vi "VNA Calibration - SParam.vi"(8 "error in":errorcluster, 10 "RFmxVNA Settings":T1={"Resource Name"="", "vCal Name"="", "RFmxVNA Calset Enable"=FALSE, "RFmxVNA Calset Interpolation"=FALSE, "Calset File Path"="", "RFmxVNA attenuation mode"=enum."s2p File", "RFmxVNA Port1 s2p file path"="", "RFmxVNA Port1 s-parameters orientation"=enum."Port1 Towards DUT", "RFmxVNA Port1 Power Compensation"=FALSE, "RFmxVNA Port2 s2p file path"="", "RFmxVNA Port2 s-parameters orientation"=enum."Port1 Towards DUT", "RFmxVNA Port2 Power Compensation"=FALSE, "Port1 Power Level (dBm)"=0.0, "Port1 Test Receiver Attenuation (dB)"=0.0, "Port2 Power Level (dBm)"=0.0, "Port2 Test Receiver Attenuation (dB)"=0.0, "IF Bandwidth (Hz)"=0.0, "Frequency Sweep"={"Start Frequency (Hz)"=4000000000.0, "Stop Frequency (Hz)"=26000000000.0, "Number of Points"=200}} {"Frequency Sweep"."Stop Frequency (Hz)" format="%.3p"; "Frequency Sweep"."Start Frequency (Hz)" format="%.3p"; "IF Bandwidth (Hz)" format="%.2p"; "Port2 Test Receiver Attenuation (dB)" format="%.2f"; "Port2 Power Level (dBm)" format="%.2f"; "Port1 Test Receiver Attenuation (dB)" format="%.2f"; "Port1 Power Level (dBm)" format="%.2f"}, 11 "RFmxVNA Session in":refnum<k21>) -> (0 "error out":errorcluster, 2 "VNA Status":string, 3 "RFmxVNA Session out":refnum<k21>)   [LabVIEW 2023]
uses:
  Controls/RFmxVNA Config - SParam.ctl
  <resource>/objmgr/RFmxVNA.rc
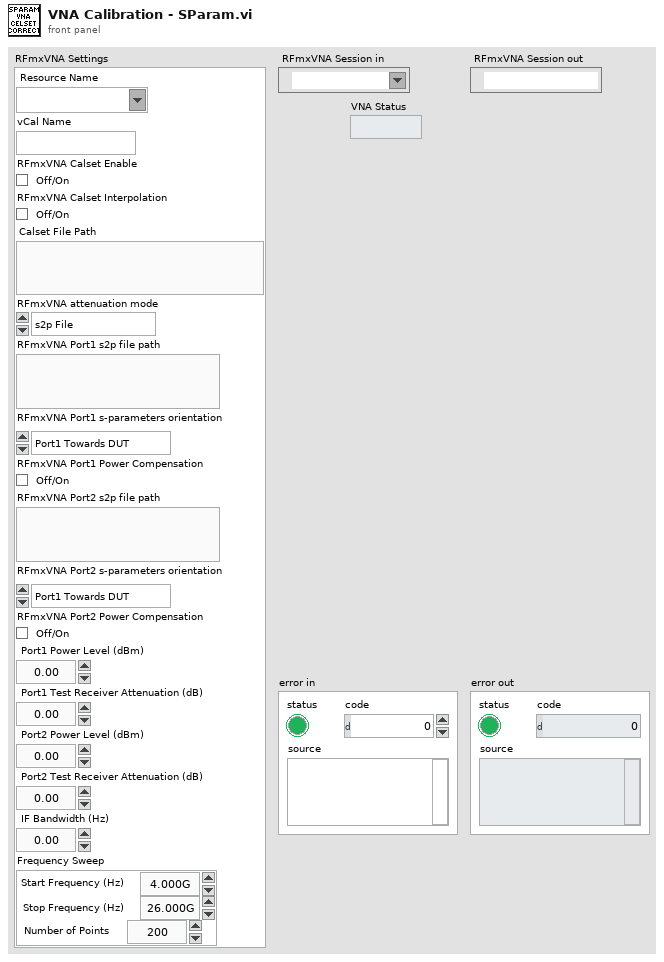
[diagram p1: front panel]
types:
  T1 = typedef "RFmxVNA Config - SParam.ctl" = cluster{"Resource Name":refnum<k15>, "vCal Name":string, "RFmxVNA Calset Enable":bool, "RFmxVNA Calset Interpolation":bool, "Calset File Path":string, "RFmxVNA attenuation mode":enum32{"<None>", "s2p File"}, "RFmxVNA Port1 s2p file path":string, "RFmxVNA Port1 s-parameters orientation":enum32{"Port1 Towards DUT", "Port2 Towards DUT"}, "RFmxVNA Port1 Power Compensation":bool, "RFmxVNA Port2 s2p file path":string, "RFmxVNA Port2 s-parameters orientation":enum32{"Port1 Towards DUT", "Port2 Towards DUT"}, "RFmxVNA Port2 Power Compensation":bool, "Port1 Power Level (dBm)":dbl, "Port1 Test Receiver Attenuation (dB)":dbl, "Port2 Power Level (dBm)":dbl, "Port2 Test Receiver Attenuation (dB)":dbl, "IF Bandwidth (Hz)":dbl, "Frequency Sweep":cluster{"Start Frequency (Hz)":dbl, "Stop Frequency (Hz)":dbl, "Number of Points":i32}}
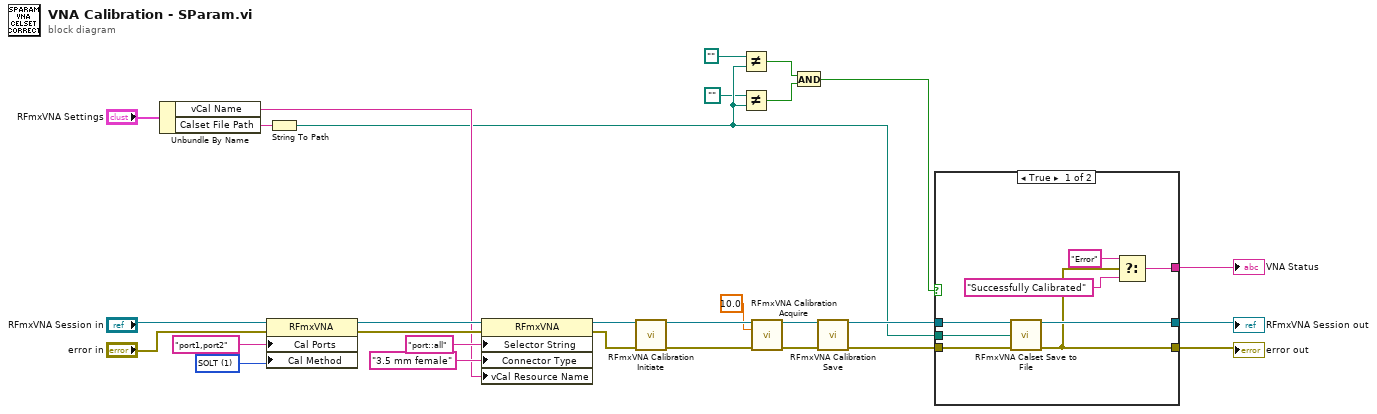
[diagram p0: block diagram]
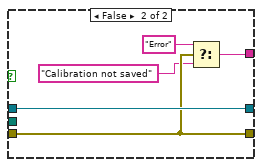
[diagram p2: hidden frame]
diagram:
  w15 = 1 items=["SOL", "SOLT", "TRL"] ("Cal Method")
  n1 = Unbundle By Name("RFmxVNA Settings") -> ("vCal Name"=w8:string, "Calset File Path"=w28:string)
  n2 = property class="RFmxVNA"(reference="RFmxVNA Session in", error in="error in", "Cal Ports"="port1,port2" ("Calibration Ports"), "Cal Method"=w15) -> (reference out=w21:refnum<k21>, error out=w20:errorcluster)
  n3 = String To Path(string=w28) -> (path=w6:path)
  n4 = property class="RFmxVNA"(reference=w21, error in=w20, "Selector String"="port::all", "Connector Type"="3.5 mm female", "vCal Resource Name"=w8) -> (reference out=w16:refnum<k21>, error out=w17:errorcluster)
  n5 = call <vilib>:"RFmxVNA Calibration Initiate.vi"("Instrument Handle In"=w16, "error in (no error)"=w17) -> ("Instrument Handle Out"=w25:refnum<k21>, "error out"=w27:errorcluster)  [unwired: 12 in]
  n6 = Not Equal?(x=path "", y=w6) -> (x != y?=w4:bool)
  n7 = Not Equal?(x=path "", y=w6) -> (x != y?=w3:bool)
  n8 = call <vilib>:"RFmxVNA Calibration Acquire.vi"("Instrument Handle In"=w25, "Timeout (s)"=10.0, "error in (no error)"=w27) -> ("Instrument Handle Out"=w24:refnum<k21>, "error out"=w26:errorcluster)  [unwired: 11 in]
  n9 = And(x=w4, y=w3) -> (x .and. y?=w2:bool)
  n10 = call <vilib>:"RFmxVNA Calibration Save.vi"("Instrument Handle In"=w24, "error in (no error)"=w26) -> ("Instrument Handle Out"=w23:refnum<k21>, "error out"=w22:errorcluster)  [unwired: 12 in]
  n11 = case shown="True" w2 {
    tunnel: w23 -> [w37 w42]
    tunnel: w22 -> [w36 w41]
    tunnel: [w34 w42] -> w12
    tunnel: [w33 w41] -> w11
    tunnel: w6 -> [w35 _]
    tunnel: [w30 w38] -> w1
    frame True {
      n12 = call <vilib>:"RFmxVNA Calset Save to File.vi"("Instrument Handle In"=w37, "Calset File Path"=w35, "error in (no error)"=w36) -> ("Instrument Handle Out"=w34:refnum<k21>, "error out"=w33:errorcluster)  [unwired: 11 in]
      n13 = Select(t="Error", s=w33, f="Successfully Calibrated") -> (s? t:f=w30:string)
    }
    frame False {
      n14 = Select(t="Error", s=w41, f="Calibration not saved") -> (s? t:f=w38:string)
    }
  }
  "error out" <- w11
  "RFmxVNA Session out" <- w12
  "VNA Status" <- w1
